vi "Initialize From File.vi"(0 "Export in":refnum<class "Export.lvclass">) -> (4 "Export out":refnum<class "Export.lvclass">)   [LabVIEW 2017, in "CL_G3_VIComponentBuilder.lvlib" / "Export.lvclass"]
doc: "Initializes the class from the configuration file."
uses:
  Export.lvclass
  Export.lvclass/Export.ctl
  Accessors/Read Export Config File.vi
  Accessors/Read Component Root path.vi
  Accessors/Write Commit behavior.vi
  Accessors/Write Export Build Specification.vi
  Accessors/Write Component Export Dir.vi
  Accessors/Write Install Built Dependencies During Build.vi
  Accessors/Write Uninstall Built Dependencies During Clean.vi
  Accessors/Write Export Operation Errors.vi
  Accessors/Read Export Operation Errors.vi
  <vilib>/Utility/libraryn.llb/Check if File or Folder Exists.vi
  <vilib>/Utility/error.llb/Error Cluster From Error Code.vi
  <vilib>/Utility/file.llb/Is Path and Not Empty.vi
  <vilib>/Utility/config.llb/NI_LVConfig.lvlib
  Commit Behavior/Commit/Commit.lvclass
  CL_G3_VIComponentBuilder.lvlib
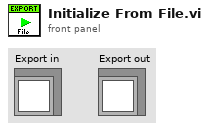
[diagram p1: front panel]
types:
  T1 = cluster{"Export Build Specification File":path, "Commit Behavior Config File":path, "Install Built Dependencies During Build":bool, "Uninstall Built Dependencies During Clean":bool}
  T2 = typedef "NI_LVConfig.lvlib/Config Data RefNum.ctl" = refnum<k1>
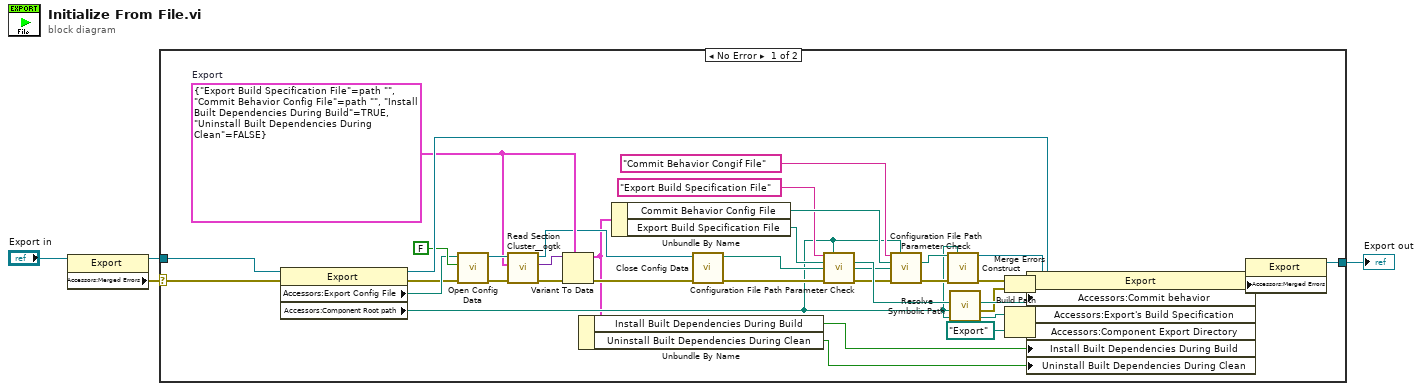
[diagram p0: block diagram]
diagram:
  n1 = property class="Export"(reference="Export in") -> (reference out=w1:refnum<class "Export.lvclass">, "Accessors:Merged Errors"=w2:errorcluster)  [unwired: 1 in, 1 out]
  n2 = case shown="No Error" w2 {
    selector: w2 -> [w25 _]
    tunnel: [w15 w43] -> w4
    tunnel: w1 -> [w42 w43]
    frame No Error {
      w36 = T1 {"Export Build Specification File"=path "", "Commit Behavior Config File"=path "", "Install Built Dependencies During Build"=TRUE, "Uninstall Built Dependencies During Clean"=FALSE}  # Export
      n3 = property class="Export"(reference=w42, error in=w25) -> (reference out=w41:refnum<class "Export.lvclass">, error out=w24:errorcluster, "Accessors:Export Config File"=w38:path, "Accessors:Component Root path"=w8:path)
      n4 = call <vilib>:"Open Config Data.vi"("error in (no error)"=w24, "create file if necessary (T)"=FALSE, "configuration file path"=w38) -> ("error out"=w35:errorcluster, "refnum"=w39:T2)  [unwired: 6 in, 1 out]
      n5 = call <userlib>:"Read Section Cluster__ogtk.vi"("error in (no error)"=w35, "Section Formatted Cluster Type"=w36, "refnum"=w39) -> ("error out"=w34:errorcluster, "Section Formatted Cluster"=w37:variant, "dup refnum"=w29:T2)  [unwired: 4 in, 2 out]
      n6 = Variant To Data(error in=w34, type=w36, Variant=w37) -> (data=w7:T1, error out=w30:errorcluster)
      n7 = Unbundle By Name(w7) -> ("Install Built Dependencies During Build"=w6:bool, "Uninstall Built Dependencies During Clean"=w5:bool)
      n8 = Unbundle By Name(w7) -> ("Commit Behavior Config File"=w33:path, "Export Build Specification File"=w28:path)
      n9 = call <vilib>:"Close Config Data.vi"("error in (no error)"=w30, "refnum"=w29) -> ("error out"=w23:errorcluster, "file path"=w21:path)  [unwired: 8 in]
      n10 = call "Configuration File Path Parameter Check.vi"("Parameter Name"="Export Build Specification File", "Component Root Path"=w8, "Specified Path in Configuration File"=w28, "Configuration File Path"=w21, "error in (no error)"=w23) -> ("dup Specified Path in Configuration File"=w26:path, "dup Configuration File Path"=w20:path, "error out"=w22:errorcluster)  [unwired: 8 in]
      n11 = call "Configuration File Path Parameter Check.vi"("Parameter Name"="Commit Behavior Congif File", "Component Root Path"=w8, "Specified Path in Configuration File"=w33, "Configuration File Path"=w20, "error in (no error)"=w22) -> ("dup Specified Path in Configuration File"=w31:path, "error out"=w18:errorcluster)  [unwired: 8 in, 1 out]
      n12 = call "Construct.vi"("Commit Behavior Config File"=w31, "Component Root Path"=w8, "error in (no error)"=w18) -> ("Commit out"=w19:refnum<class "Commit.lvclass">, "error out"=w17:errorcluster)  [unwired: 11 in]
      n13 = call "Resolve Symbolic Path.vi"("Component Root Path"=w8, "Path In"=w26) -> ("error out"=w9:errorcluster, "Path Out"=w12:path)  [unwired: 8 in]
      n14 = Merge Errors(w17, w9) -> (w10:errorcluster)
      n15 = Build Path(base path=w8, name or relative path=path "Export" ("VIPB Path")) -> (appended path=w11:path)
      n16 = property class="Export"(reference=w41, error in=w10, "Accessors:Commit behavior"=w19, "Accessors:Export's Build Specification"=w12, "Accessors:Component Export Directory"=w11, "Install Built Dependencies During Build"=w6, "Uninstall Built Dependencies During Clean"=w5) -> (reference out=w16:refnum<class "Export.lvclass">, error out=w14:errorcluster)
      n17 = property class="Export"(reference=w16, "Accessors:Merged Errors"=w14) -> (reference out=w15:refnum<class "Export.lvclass">)  [unwired: 1 in, 1 out]
    }
    frame Error {
    }
  }
  "Export out" <- w4
